vi "writer.vi"() -> ()   [LabVIEW 2020]
uses:
  <vilib>/measure/madcrms.llb/Basic Averaged DC-RMS for 1 Chan.vi
  <vilib>/measure/NI_MAPro.lvlib
panel:
  in  "Path":path
  out "time signal":waveform(dbl)
  in  "stop":bool
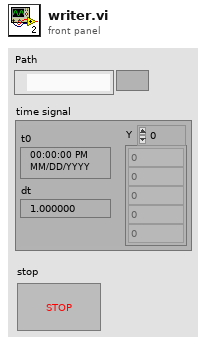
[diagram p1: front panel]
types:
  T1 = enum16{"open", "open or create", "create or replace", "create", "open (read-only)"}
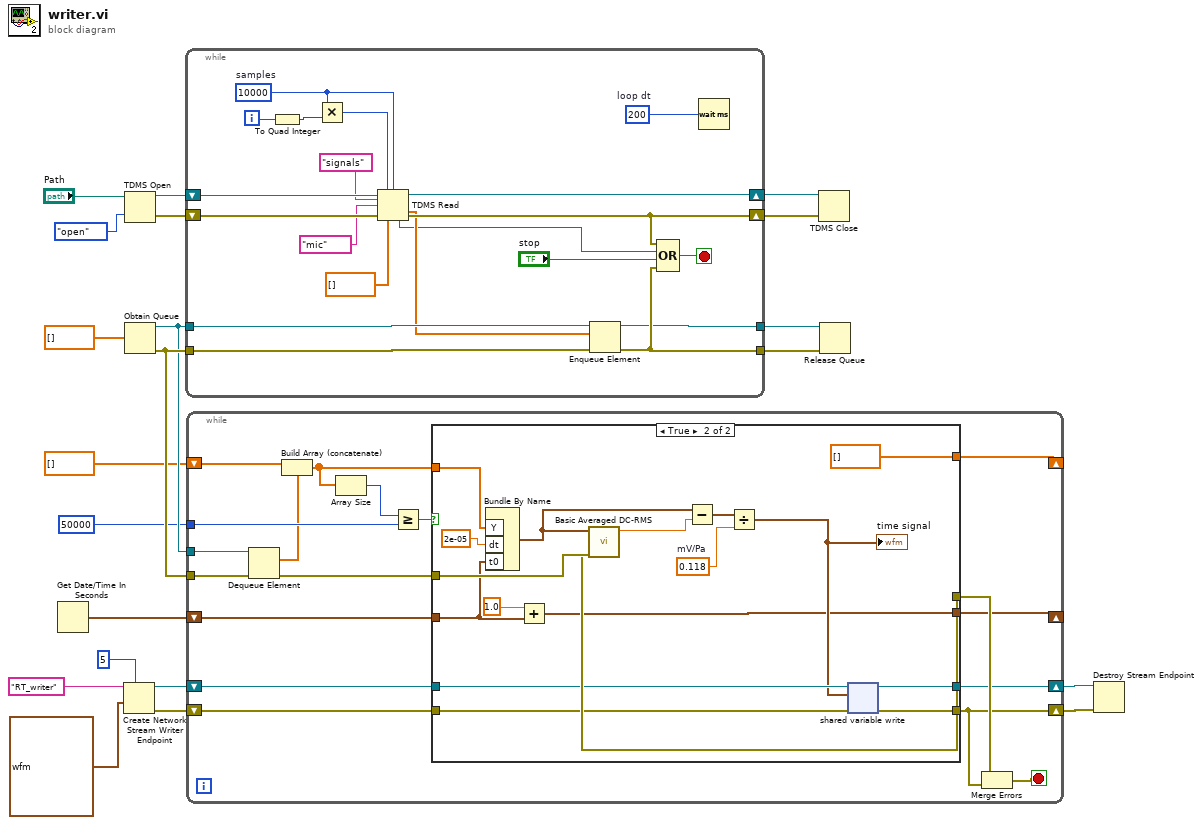
[diagram p0: block diagram]
diagram:
  n1 = Get Date/Time In Seconds() -> (seconds since 1Jan1904=w1:timestamp)
  n2 = Create Network Stream Writer Endpoint(7:5 ("writer buffer size"), 9:waveform(dbl) {"t0"=timestamp(0 s since 1904-01-01), "dt"=1.0, "Y"=[]} ("time signal"), 11:"RT_writer" ("writer name")) -> (0:w4:errorcluster, 3:w5:refnum<k21>)  [unwired: 4 in]
  n3 = TDMS Open(10:T1."open" ("operation (0:open)"), 11:"Path") -> (0:w19:errorcluster, 3:w21:refnum<k34>)  [unwired: 5 in]
  n4 = Obtain Queue(element data type=dbl[] []) -> (queue out=w12:refnum<queue>, error out=w13:errorcluster)  [unwired: 4 in, 1 out]
  n5 = while {
    shift-right: [w37] -> w20
    shift-left: w21 -> [w38]
    shift-right: [w31] -> w18
    shift-left: w19 -> [w36]
    tunnel: w13 -> [w30]
    tunnel: [w29] -> w16
    tunnel: w12 -> [w27]
    tunnel: [w26] -> w14
    i -> [w41]
    stop <- w28 stop-if-true
    w39 = 200  # loop dt
    w34 = 10000  # samples
    n6 = To Quad Integer(1:w41) -> (0:w40:i64)
    n7 = Multiply(x=w34, y=w40) -> (x*y=w35:i64)
    n8 = TDMS Read(0:w38, 1:w35, 2:w34, 5:"signals", 7:"mic", 11:w36, 12:dbl[] []) -> (4:w37:refnum<k34>, 10:w24:dbl[], 14:w22:bool, 15:w31:errorcluster)  [unwired: 1 in, 2 out]
    n9 = Enqueue Element(queue=w27, element=w24, error in (no error)=w30) -> (queue out=w26:refnum<queue>, error out=w29:errorcluster)  [unwired: 1 in, 1 out]
    n10 = Compound Arithmetic op=OR(w31, w22, "stop", w29) -> (w28:bool)
    n11 = Wait (ms)(milliseconds to wait=w39) -> ()  [unwired: 1 out]
  }
  n12 = while {
    tunnel: w13 -> [w59]
    tunnel: w12 -> [w58]
    shift-right: [w54] -> _
    shift-left: dbl[] [] -> [w55]
    shift-right: [w50] -> w7
    shift-left: w5 -> [w48]
    shift-right: [w49] -> w6
    shift-left: w4 -> [w47]
    tunnel: 50000 -> [w45]
    shift-right: [w42] -> _
    shift-left: w1 -> [w43]
    stop <- w52 stop-if-true
    n13 = Dequeue Element(queue=w58, error in (no error)=w59) -> (element=w44:dbl[], error out=w53:errorcluster)  [unwired: 1 in, 2 out]
    n14 = Build Array (concatenate)(w55, w44) -> (w46:dbl[])
    n15 = Array Size(array=w46) -> (size(s)=w56:i32)
    n16 = Greater Or Equal?(x=w56, y=w45) -> (x >= y?=w57:bool)
    n17 = case shown="True" w57 {
      tunnel: w46 -> [w64 w81]
      tunnel: [w64 dbl[] []] -> w54
      tunnel: w53 -> [w61 w75]
      tunnel: [w61 w74] -> w51
      tunnel: [w63 w73] -> w50
      tunnel: [w62 w72] -> w49
      tunnel: w48 -> [w63 w71]
      tunnel: w47 -> [w62 w70]
      tunnel: w43 -> [w60 w68]
      tunnel: [w60 w66] -> w42
      frame False {
      }
      frame True {
        w65 = 0.118  # mV/Pa
        n18 = Bundle By Name("Y"=w81, "dt"=2e-05, "t0"=w68) -> (w78:waveform(dbl))  [unwired: 1 in]
        n19 = Add(x=1.0, y=w68) -> (x+y=w66:timestamp)
        n20 = call-poly <vilib>:"Basic Averaged DC-RMS.vi"("error in (no error)"=w75, "signal in"=w78) -> ("error out"=w74:errorcluster, "DC value"=w79:dbl)  [unwired: 6 in, 2 out]
        n21 = Subtract(x=w78, y=w79) -> (x-y=w76:waveform(dbl))
        n22 = Divide(x=w76, y=w65) -> (x/y=w69:waveform(dbl))
        "time signal" <- w69
        n23 = shared-variable-write(w71, w70, w69) -> (w73:refnum<k21>, w72:errorcluster)  [unwired: 1 in, 1 out]
      }
    }
    n24 = Merge Errors(w51, w49) -> (w52:errorcluster)
  }
  n25 = TDMS Close(8:w18, 11:w20) -> ()  [unwired: 2 out]
  n26 = Release Queue(queue=w14, error in (no error)=w16) -> ()  [unwired: 1 in, 3 out]
  n27 = Destroy Stream Endpoint(8:w6, 11:w7) -> ()  [unwired: 1 out]
